vi "clear_buffers.vi"(8 "error in (no error)":errorcluster, 11 "FPGAWrapperDL090211Galvo in":refnum<class "FPGAWrapperDL090211Galvo_grabber.lvclass">) -> (0 "error out":errorcluster, 3 "FPGAWrapperDL090211Galvo out":refnum<class "FPGAWrapperDL090211Galvo_grabber.lvclass">)   [LabVIEW 2010, in "FPGAWrapperDL090211Galvo_grabber.lvclass"]
uses:
  FPGAWrapperDL090211Galvo_grabber.lvclass
  type definitions/command_enum.ctl
  class_data.vi
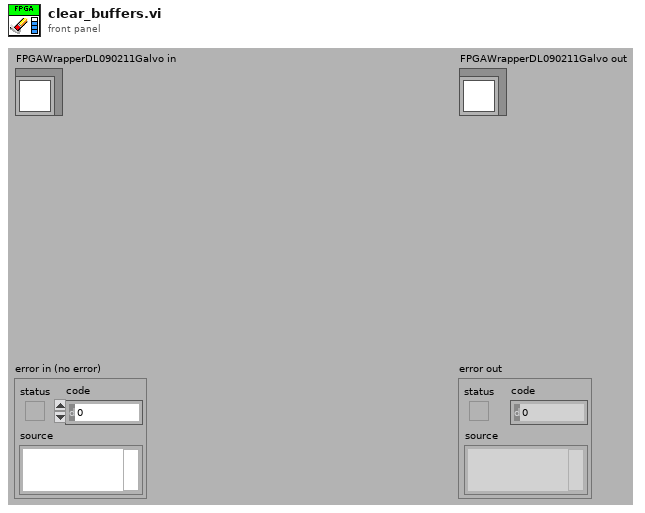
[diagram p1: front panel]
types:
  T1 = typedef "command_enum.ctl" = enum16{"NULL", "update", "start", "stop", "reset", "shut-down"}
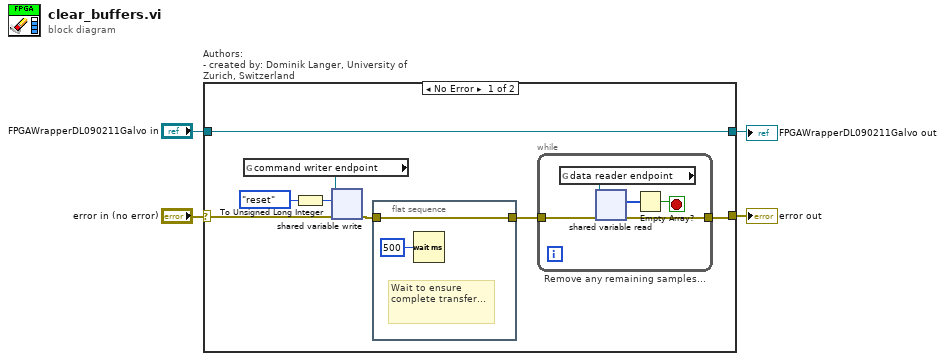
[diagram p0: block diagram]
diagram:
  n1 = case "Authors: \n- created by: Dominik Langer, University of Zurich, Switzerland" shown="No Error" "error in (no error)" {
    selector: "error in (no error)" -> [w10 w20]
    tunnel: "FPGAWrapperDL090211Galvo in" -> [w9 w21]
    tunnel: [w9 w21] -> w2
    tunnel: [w7 w20] -> w1
    frame No Error {
      n2 = global read "class_data.vi" "command writer endpoint"() -> (w8:refnum<k21>)
      n3 = To Unsigned Long Integer(number=command_enum."reset" ("command")) -> (unsigned 32bit integer=w12:u32)
      n4 = shared-variable-write(w8, w10, w12) -> (w6:errorcluster)  [unwired: 1 in, 2 out]
      n5 = flat-sequence {
        tunnel: w6 -> [w19]
        tunnel: [w19] -> w5
        frame #0 {
          # "Wait to ensure complete transfer..."
          n6 = Wait (ms)(milliseconds to wait=u32 500) -> ()  [unwired: 1 out]
        }
      }
      n7 = while "Remove any remaining samples..." {
        tunnel: [w17] -> w7
        tunnel: w5 -> [w15]
        stop <- w13 stop-if-true
        n8 = global read "class_data.vi" "data reader endpoint"() -> (w16:refnum<k21>)
        n9 = shared-variable-read(w16, w15) -> (w17:errorcluster, w14:u64[])  [unwired: 2 in, 2 out]
        n10 = Empty Array?(array=w14) -> (empty?=w13:bool)
      }
    }
    frame Error {
    }
  }
  "error out" <- w1
  "FPGAWrapperDL090211Galvo out" <- w2
